vi "Set_Tunnel_Speed_server.vi"(4 "Tunnel Velocity m/s":dbl min=0.0 max=50.0 format="%#.3f", 5 "Rig Name":string, 6 "Mode":T1, 7 "Client Name":string="G3_3 HD") -> (0 "Error String":string, 1 "Settling Time (s)":dbl format="%.2f", 2 "Max allowable Tunnel Velocity":dbl, 3 "Valid Client":bool)   [LabVIEW 2022 SP3]
uses:
  ADAM Client/Sub VIs/ADAM Controls/Tunnel_speed_mode.ctl
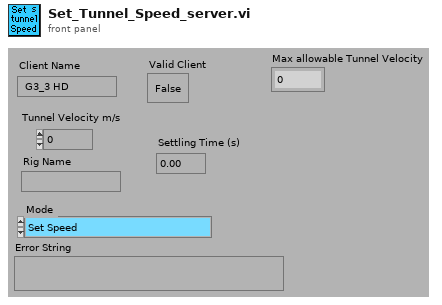
[diagram p1: front panel]
types:
  T1 = typedef "Tunnel_speed_mode.ctl" = enum16{"Set Speed", "Set Speed then wait", "Is tunnel speed allowable?"}
  T2 = typedef "Ch_description_ADAM.ctl" = cluster{"Ch Name":string, "Type":T3, "Function":T4, "Ch State":T5, "Calibration type":T6, "A":dbl, "B":dbl, "C":dbl, "D":dbl, "Comments":string, "Address":T7, "String":string, "Duty":u16}
  T3 = typedef "Module_type_ADAM.ctl" = string
  T4 = typedef "Function_ADAM.ctl" = enum16{"Analogue Input", "Digital Input", "Event counter", "Event rate", "Analogue Output", "Digital Output", "Relay Output"}
  T5 = typedef "Channel_State.ctl" = enum16{"On", "Off", "Always On", "Always Off"}
  T6 = typedef "Calib_type_ADAM.ctl" = string
  T7 = typedef "Address.ctl" = cluster{"Main":i32, "Ch.":i32, "Sub":i32, "Port Name":string}
  T8 = cluster{"Bus Bar":string, "Connected Items":string[]}
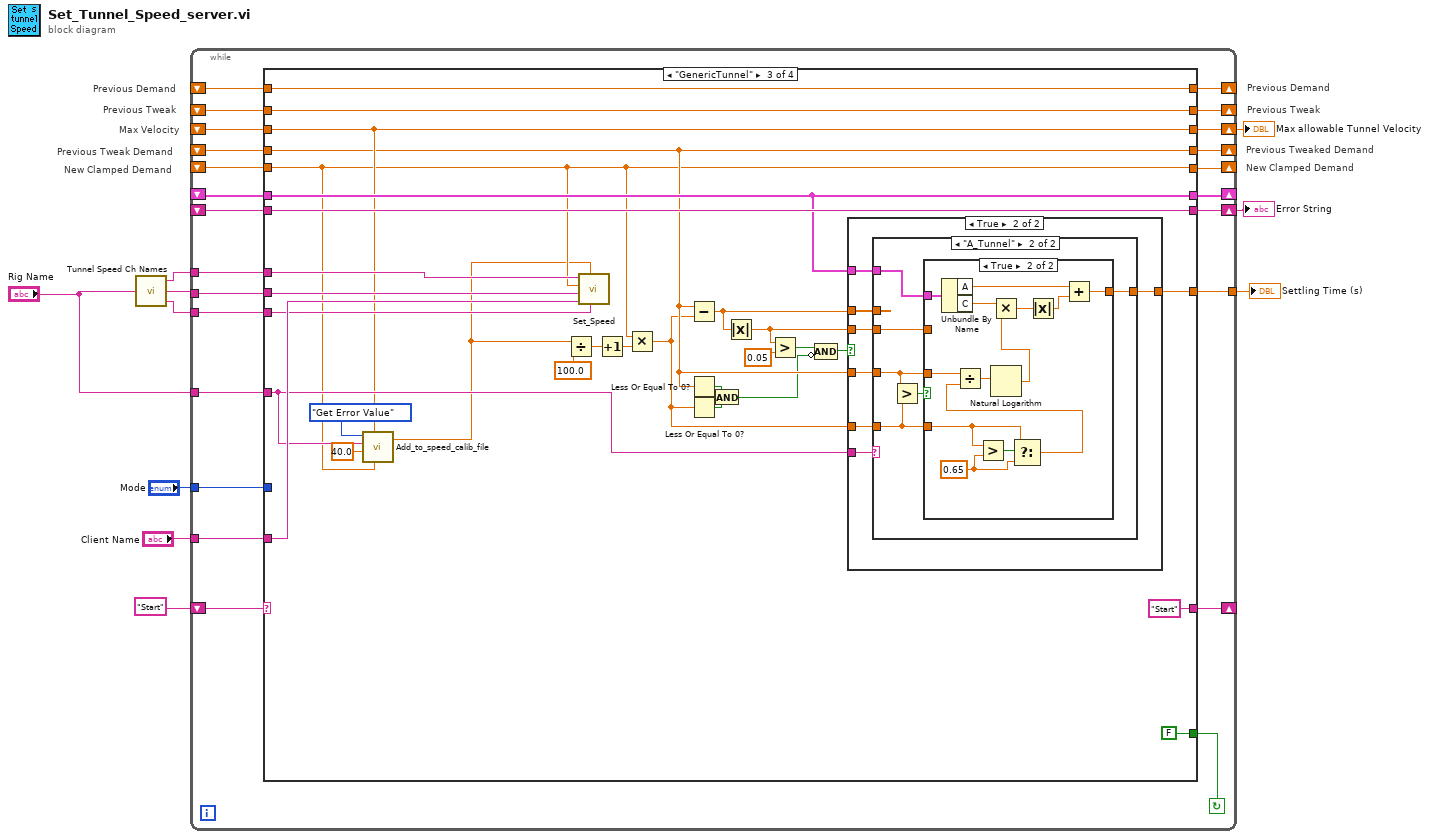
[diagram p0: block diagram]
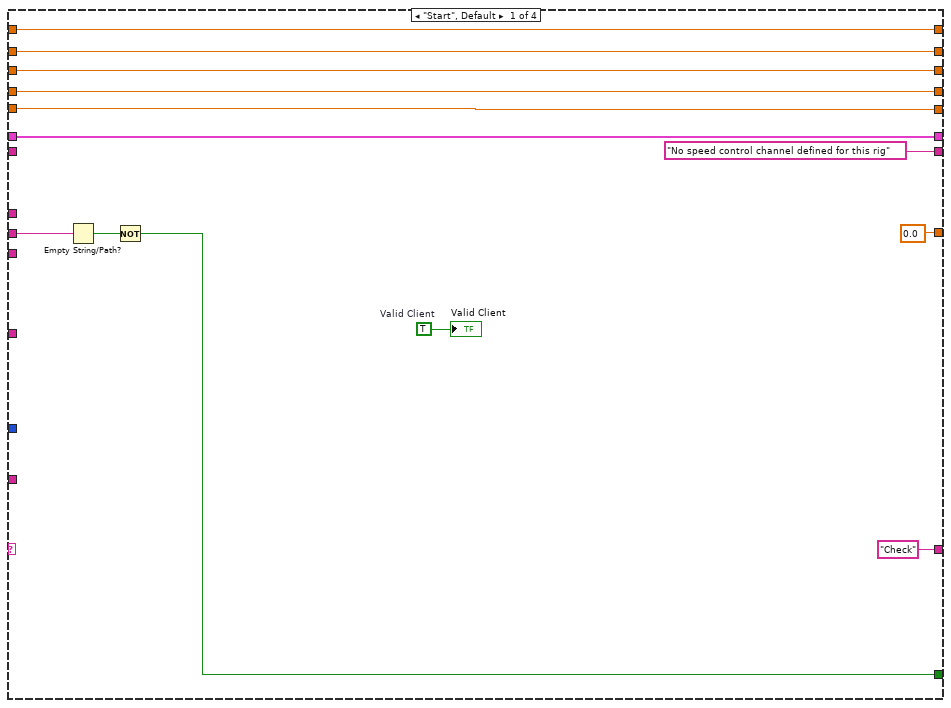
[diagram p2: hidden frame]
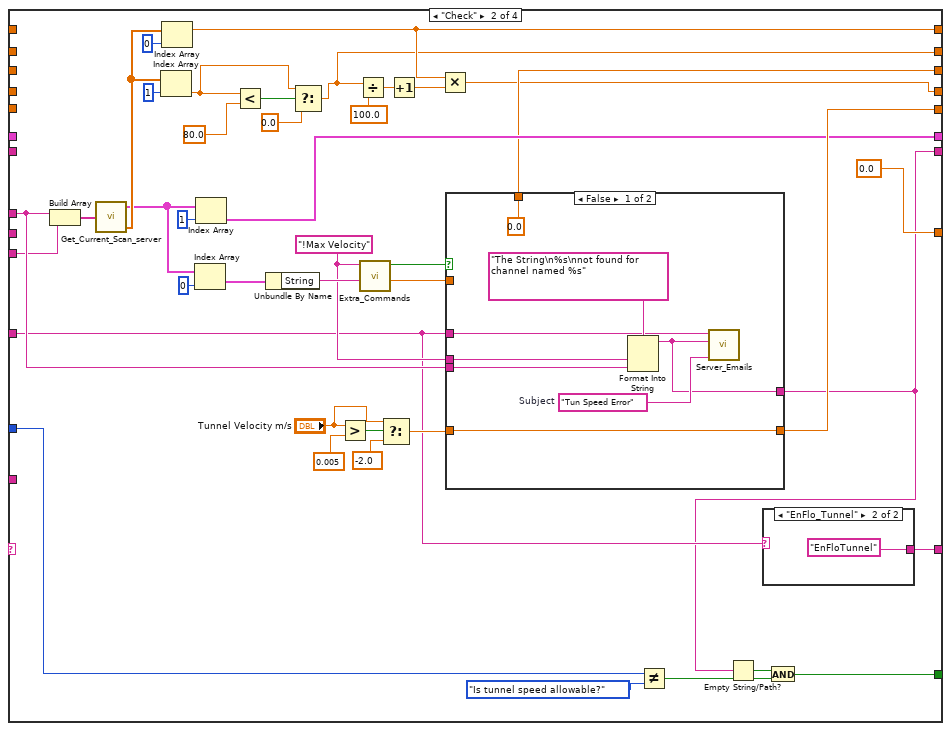
[diagram p3: hidden frame]
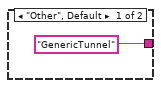
[diagram p4: hidden frame]
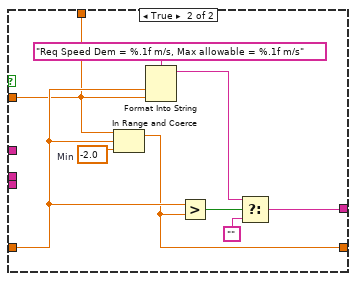
[diagram p5: hidden frame]
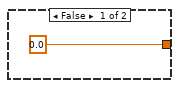
[diagram p6: hidden frame]
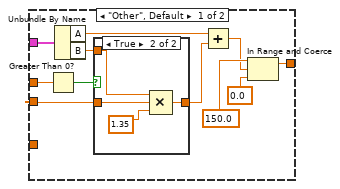
[diagram p7: hidden frame]
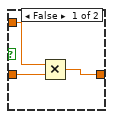
[diagram p8: hidden frame]
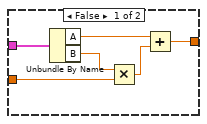
[diagram p9: hidden frame]
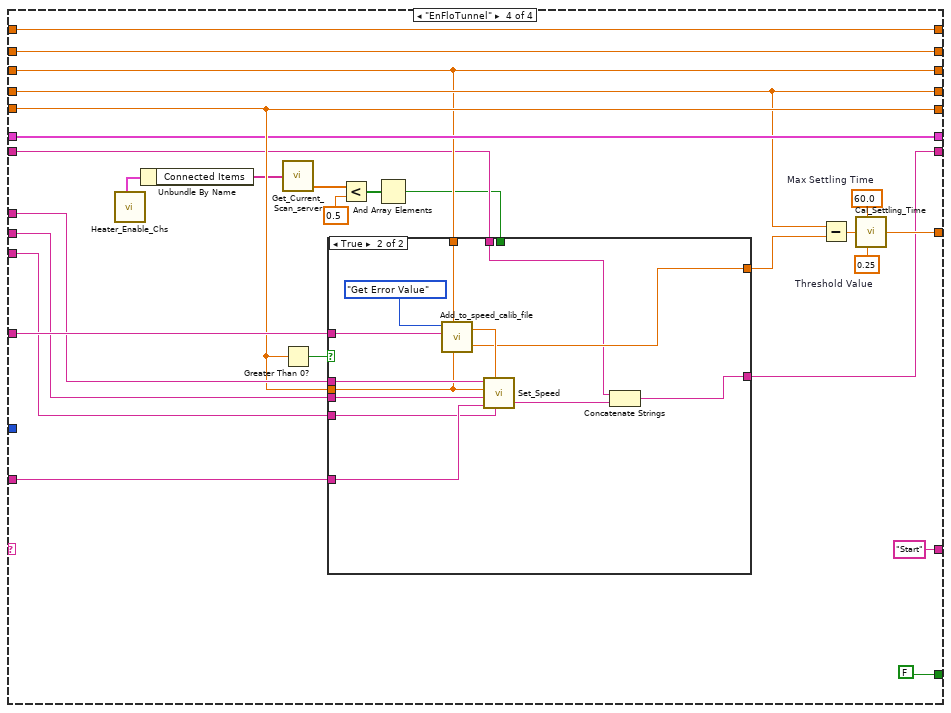
[diagram p10: hidden frame]
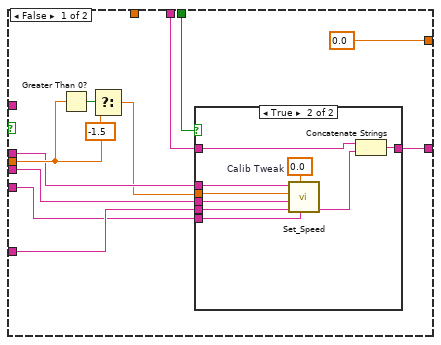
[diagram p11: hidden frame]
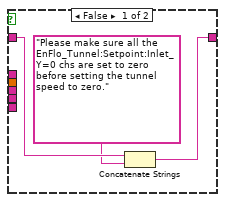
[diagram p12: hidden frame]
diagram:
  # "New Clamped Demand"
  # "Max Velocity"
  # "Previous Tweak Demand"
  # "Previous Tweak"
  # "Previous Demand"
  # "Previous Tweak"
  # "Previous Demand"
  # "Previous Tweaked Demand"
  # "New Clamped Demand"
  n1 = call "Tunnel Speed Ch Names.vi"("Rig Name"="Rig Name") -> ("Calib Tweak"=w1:string, "Dem Voltage"=w2:string, "Dem Velocity"=w3:string)  [unwired: 2 in]
  n2 = while {
    shift-left: _ -> [w17]
    shift-right: [w18] -> _
    tunnel: w1 -> [w19]
    shift-left: _ -> [w21]
    shift-right: [w20] -> _
    tunnel: [w22] -> w7
    tunnel: w2 -> [w24]
    shift-left: _ -> [w23]
    shift-right: [w27] -> w9
    shift-left: _ -> [w25]
    shift-right: [w28] -> _
    tunnel: w3 -> [w29]
    shift-left: "Start" -> [w31]
    shift-right: [w30] -> _
    tunnel: "Client Name" -> [w33]
    tunnel: "Mode" -> [w34]
    tunnel: "Rig Name" -> [w32]
    shift-right: [w16] -> w6
    shift-left: _ -> [w15]
    shift-right: [w14] -> _
    shift-left: _ -> [w12]
    shift-right: [w13] -> _
    shift-left: _ -> [w11]
    stop <- w26 continue-if-true
    n3 = case shown="\"GenericTunnel\"" w31 {
      tunnel: w25 -> [w44 _ w111 w208]
      tunnel: w34 -> [_ w79 _ _]
      tunnel: ["No speed control channel defined for this rig" w56 w133 w197] -> w27
      tunnel: w33 -> [_ _ w137 w214]
      tunnel: w32 -> [_ w72 w127 w213]
      tunnel: ["Check" w75 "Start" "Start"] -> w30
      tunnel: w29 -> [_ w83 w135 w211]
      tunnel: [w44 w81 w111 w208] -> w28
      tunnel: [w45 w55 FALSE FALSE] -> w26
      tunnel: w24 -> [w47 _ w134 w210]
      tunnel: w23 -> [_ _ w133 w198]
      tunnel: [0.0 ("Settling Time") 0.0 ("Settling Time") w130 w206] -> w22
      tunnel: w21 -> [w42 _ w123 w201]
      tunnel: [w42 w53 w123 w201] -> w20
      tunnel: w19 -> [_ w71 w131 w204]
      tunnel: [w40 w60 w129 w202] -> w18
      tunnel: w17 -> [w40 _ w129 w202]
      tunnel: [w39 w59 w126 w200] -> w16
      tunnel: w15 -> [w39 _ w126 w200]
      tunnel: [w38 w54 w117 w191] -> w14
      tunnel: [w37 w51 w112 w190] -> w13
      tunnel: w12 -> [w38 _ w117 w191]
      tunnel: w11 -> [w37 _ w112 w190]
      frame "Start", Default {
        w36 = TRUE  # Valid Client
        n4 = Empty String/Path?(string/path=w47) -> (empty?=w46:bool)
        n5 = Not(x=w46) -> (.not. x?=w45:bool)
        "Valid Client" <- w36
      }
      frame "Check" {
        w84 = "!Max Velocity" ("Command")
        n6 = Build Array(w83, w71) -> (w88:string[])
        n7 = call "Get_Current_Scan_server.vi"("Desired Channels"=w88) -> ("Ch Description Array"=w61:T2[], "Numerical Values"=w69:dbl[])  [unwired: 1 out]
        n8 = Index Array(array=w69, index=1 ("Index")) -> (element=w48:dbl)
        n9 = Index Array(array=w69, index=0 ("Index")) -> (element=w54:dbl)
        n10 = Index Array(array=w61, index=0 ("Index")) -> (element=w63:T2)
        n11 = Index Array(array=w61, index=1 ("Index")) -> (element=w60:T2)
        n12 = Less?(x=w48, y=80.0 ("f")) -> (x < y?=w49:bool)
        n13 = Unbundle By Name(w63) -> ("String"=w86:string)
        n14 = Select(t=w48, s=w49, f=0.0) -> (s? t:f=w51:dbl)
        n15 = Greater?(x="Tunnel Velocity m/s", y=0.005) -> (0:w78:bool)
        n16 = Divide(x=w51, y=100.0) -> (x/y=w67:dbl)
        n17 = call "Extra_Commands.vi"("String to Search"=w86, "Command"=w84) -> ("Numeric Value"=w82:dbl, "Command Found"=w85:bool)  [unwired: 1 in, 3 out]
        n18 = Select(t="Tunnel Velocity m/s", s=w78, f=-2.0 ("t")) -> (s? t:f=w76:dbl)
        n19 = Increment(x=w67) -> (x+1=w66:dbl)
        n20 = Multiply(x=w54, y=w66) -> (x*y=w53:dbl)
        n21 = case shown="False" w85 {
          tunnel: w72 -> [w92 _]
          tunnel: w84 -> [w97 _]
          tunnel: w83 -> [w96 _]
          tunnel: w82 -> [_ w99]
          tunnel: w76 -> [w94 w101]
          tunnel: [w94 w100] -> w81
          tunnel: [w93 w103] -> w56
          tunnel: [0.0 ("Numeric Value") w99] -> w59
          frame False {
            w98 = "Tun Speed Error"  # Subject
            n22 = Format Into String(format string="The String\n%s\nnot found for channel named %s" ("Format String"), w97, w96) -> (resulting string=w93:string)  [unwired: 2 in, 1 out]
            n23 = call "Server_Emails.vi"("Client Name Contains"=w92, "Message"=w93, "Subject"=w98) -> ()  [unwired: 2 in, 3 out]
          }
          frame True {
            w107 = -2.0  # Min
            n24 = In Range and Coerce(upper limit=w99, x=w101, lower limit=w107) -> (coerced(x)=w100:dbl)  [unwired: 1 out]
            n25 = Format Into String(format string="Req Speed Dem = %.1f m/s, Max allowable = %.1f m/s", w101, w99) -> (resulting string=w105:string)  [unwired: 2 in, 1 out]
            n26 = Greater?(x=w101, y=w100) -> (0:w102:bool)
            n27 = Select(t=w105, s=w102, f="") -> (s? t:f=w103:string)
          }
        }
        n28 = Not Equal?(x=w79, y=Tunnel_speed_mode."Is tunnel speed allowable?" ("Mode")) -> (x != y?=w57:bool)
        n29 = Empty String/Path?(string/path=w56) -> (empty?=w58:bool)
        n30 = case shown="\"EnFlo_Tunnel\"" w72 {
          tunnel: ["GenericTunnel" "EnFloTunnel"] -> w75
          frame "Other", Default {
          }
          frame "EnFlo_Tunnel" {
          }
        }
        n31 = And(x=w58, y=w57) -> (x .and. y?=w55:bool)
      }
      frame "GenericTunnel" {
        n32 = call "Add_to_speed_calib_file.vi"("Desired Velocity"=w111, "Max Velocity"=w126, "Max % Tweak allowable"=40.0, "Rig Name"=w127, "Mode"=enum16{"Add Row", "Get Error Value"}."Get Error Value") -> ("Calib Tweak %"=w108:dbl)  [unwired: 1 in, 1 out]
        n33 = Divide(x=w108, y=100.0) -> (x/y=w115:dbl)
        n34 = call "Set_Speed.vi"("Channel Name (Calib Tweak)"=w131, "Calib Tweak"=w108, "Client Name"=w137, "Channel Name (Volts/Amps)"=w134, "Demanded Velocity"=w111, "Channel Name (Velocity)"=w135) -> ()  [unwired: 1 in, 4 out]
        n35 = Increment(x=w115) -> (x+1=w116:dbl)
        n36 = Multiply(x=w111, y=w116) -> (x*y=w113:dbl)
        n37 = Subtract(x=w123, y=w113) -> (x-y=w128:dbl)
        n38 = Less Or Equal To 0?(x=w123) -> (x <= 0?=w119:bool)
        n39 = Less Or Equal To 0?(x=w113) -> (x <= 0?=w120:bool)
        n40 = And(x=w119, y=w120) -> (x .and. y?=w118:bool)
        n41 = Absolute Value(x=w128) -> (abs(x)=w125:dbl)
        n42 = Greater?(x=w125, y=0.05) -> (0:w122:bool)
        n43 = Compound Arithmetic op=AND(w122, invert w118) -> (w121:bool)
        n44 = case shown="True" w121 {
          tunnel: [0.0 ("Max") w145] -> w130
          tunnel: w129 -> [_ w144]
          tunnel: w128 -> [_ w143]
          tunnel: w123 -> [_ w142]
          tunnel: w113 -> [_ w141]
          tunnel: w127 -> [_ w140]
          tunnel: w125 -> [_ w139]
          frame False {
          }
          frame True {
            n45 = case shown="\"A_Tunnel\"" w140 {
              tunnel: w144 -> [w156 w168]
              tunnel: w143 -> [w151 _]
              tunnel: w139 -> [w147 w169]
              tunnel: [w146 w167] -> w145
              tunnel: w142 -> [_ w165]
              tunnel: w141 -> [_ w166]
              frame "Other", Default {
                n46 = Greater Than 0?(x=w151) -> (x > 0?=w150:bool)
                n47 = Unbundle By Name(w156) -> ("A"=w155:dbl, "B"=w149:dbl)
                n48 = case shown="True" w150 {
                  tunnel: [w159 w160] -> w148
                  tunnel: w149 -> [w158 w163]
                  tunnel: w147 -> [w157 w162]
                  frame False {
                    n49 = Multiply(x=w158, y=w157) -> (x*y=w159:dbl)
                  }
                  frame True {
                    n50 = Compound Arithmetic op=MULTIPLY(w163, w162, 1.35 ("Min")) -> (w160:dbl)
                  }
                }
                n51 = Add(x=w155, y=w148) -> (x+y=w152:dbl)
                n52 = In Range and Coerce(upper limit=150.0 ("Max"), x=w152, lower limit=0.0 ("Min")) -> (coerced(x)=w146:dbl)  [unwired: 1 out]
              }
              frame "A_Tunnel" {
                n53 = Greater?(x=w165, y=w166) -> (0:w164:bool)
                n54 = case shown="True" w164 {
                  tunnel: w169 -> [w171 _]
                  tunnel: w168 -> [w175 w188]
                  tunnel: [w170 w180] -> w167
                  tunnel: w165 -> [_ w186]
                  tunnel: w166 -> [_ w178]
                  frame False {
                    n55 = Unbundle By Name(w175) -> ("A"=w174:dbl, "B"=w172:dbl)
                    n56 = Multiply(x=w172, y=w171) -> (x*y=w173:dbl)
                    n57 = Add(x=w174, y=w173) -> (x+y=w170:dbl)
                  }
                  frame True {
                    w177 = 0.65 ("y")
                    n58 = Unbundle By Name(w188) -> ("A"=w181:dbl, "C"=w184:dbl)
                    n59 = Greater?(x=w178, y=w177) -> (0:w179:bool)
                    n60 = Select(t=w178, s=w179, f=w177) -> (s? t:f=w176:dbl)
                    n61 = Divide(x=w186, y=w176) -> (x/y=w187:dbl)
                    n62 = Natural Logarithm(1:w187) -> (0:w185:dbl)
                    n63 = Multiply(x=w184, y=w185) -> (x*y=w183:dbl)
                    n64 = Absolute Value(x=w183) -> (abs(x)=w182:dbl)
                    n65 = Add(x=w181, y=w182) -> (x+y=w180:dbl)
                  }
                }
              }
            }
          }
        }
      }
      frame "EnFloTunnel" {
        w207 = 0.25  # Threshold Value
        w199 = 60.0  # Max Settling Time
        n66 = call "Heater_Enable_Chs.vi"() -> ("Inlet Heaters"=w196:T8)  [unwired: 4 in, 5 out]
        n67 = Unbundle By Name(w196) -> ("Connected Items"=w195:string[])
        n68 = call "Get_Current_Scan_server.vi"("Desired Channels"=w195) -> ("Numerical Values"=w194:dbl[])  [unwired: 2 out]
        n69 = Greater Than 0?(x=w208) -> (x > 0?=w215:bool)
        n70 = Less?(x=w194, y=0.5) -> (x < y?=w193:bool[])
        n71 = And Array Elements(Boolean array=w193) -> (logical AND=w192:bool)
        n72 = case shown="True" w215 {
          tunnel: w208 -> [w225 w244]
          tunnel: w211 -> [w224 w252]
          tunnel: w210 -> [w222 w251]
          tunnel: w214 -> [w221 w250]
          tunnel: w213 -> [_ w249]
          tunnel: w192 -> [w220 _]
          tunnel: [0.0 w245] -> w203
          tunnel: w204 -> [w218 w247]
          tunnel: w200 -> [_ w243]
          tunnel: w198 -> [w217 w242]
          tunnel: [w216 w240] -> w197
          frame False {
            n73 = Greater Than 0?(x=w225) -> (x > 0?=w227:bool)
            n74 = Select(t=w225, s=w227, f=-1.5 ("t")) -> (s? t:f=w223:dbl)
            n75 = case shown="True" w220 {
              tunnel: w224 -> [_ w239]
              tunnel: w223 -> [_ w238]
              tunnel: w222 -> [_ w237]
              tunnel: w221 -> [_ w236]
              tunnel: w218 -> [_ w235]
              tunnel: w217 -> [w230 w231]
              tunnel: [w228 w233] -> w216
              frame False {
                n76 = Concatenate Strings(w230, "Please make sure all the EnFlo_Tunnel:Setpoint:Inlet_Y=0 chs are set to zero before setting the tunnel speed to zero.") -> (w228:string)
              }
              frame True {
                w234 = 0.0  # Calib Tweak
                n77 = call "Set_Speed.vi"("Channel Name (Calib Tweak)"=w235, "Calib Tweak"=w234, "Client Name"=w236, "Channel Name (Volts/Amps)"=w237, "Demanded Velocity"=w238, "Channel Name (Velocity)"=w239) -> ("Errors"=w232:string)  [unwired: 1 in, 3 out]
                n78 = Concatenate Strings(w231, w232) -> (w233:string)
              }
            }
          }
          frame True {
            n79 = call "Add_to_speed_calib_file.vi"("Desired Velocity"=w244, "Max Velocity"=w243, "Rig Name"=w249, "Mode"=enum16{"Add Row", "Get Error Value"}."Get Error Value") -> ("Tweaked Demand"=w245:dbl, "Calib Tweak %"=w246:dbl)  [unwired: 2 in]
            n80 = call "Set_Speed.vi"("Channel Name (Calib Tweak)"=w247, "Calib Tweak"=w246, "Client Name"=w250, "Channel Name (Volts/Amps)"=w251, "Demanded Velocity"=w244, "Channel Name (Velocity)"=w252) -> ("Errors"=w241:string)  [unwired: 1 in, 3 out]
            n81 = Concatenate Strings(w242, w241) -> (w240:string)
          }
        }
        n82 = Subtract(x=w201, y=w203) -> (x-y=w205:dbl)
        n83 = call "Cal_Settling_Time.vi"("Max Settling Time"=w199, "Speed Tweak (m/s)"=w205, "Threshold Value"=w207) -> ("Required Settling Time"=w206:dbl)  [unwired: 2 out]
      }
    }
  }
  "Error String" <- w9
  "Settling Time (s)" <- w7
  "Max allowable Tunnel Velocity" <- w6
